vi "Heater_Setpoint_Panel.vi"() -> ()   [LabVIEW 2016]
uses:
  Heater_Setpoint.ctl
  ADAM Controls/Channel_names.ctl
  ADAM Controls/Update_scan_value.ctl
  ADAM Controls/Channel_State.ctl
panel:
  in  "Mode":u16(ring) items=["Only Show Setpoints Above 2 Deg C", "Show all Setpoints"]
  in  "Setpoints Out":T1[](array[typedef])
  out "Messages":string
  in  "OK":bool
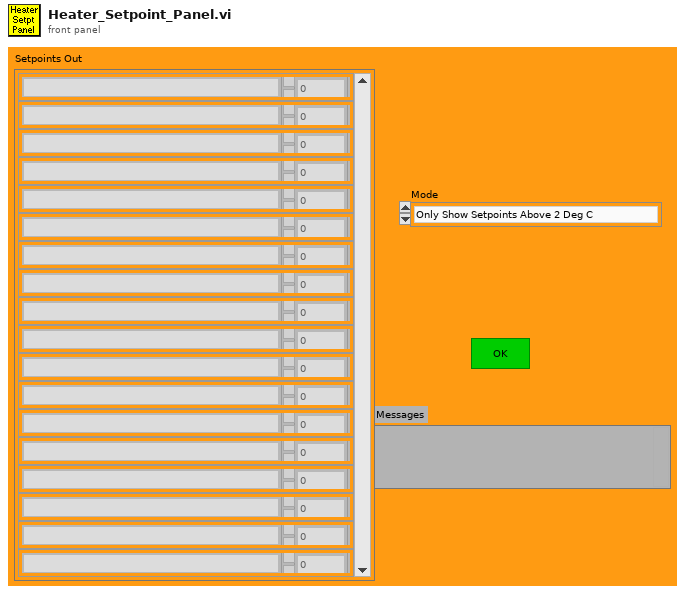
[diagram p1: front panel]
types:
  T1 = typedef "Heater_Setpoint.ctl" = cluster{"Ch Name":string, "Setpoint":dbl}
  T2 = typedef "Channel_names.ctl" = enum16{"Active Only", "Active + Off", "All Channels"}
  T3 = typedef "Update_scan_value.ctl" = cluster{"Channel Name":string, "New Value":dbl}
  T4 = typedef "Channel_State.ctl" = enum16{"On", "Off", "Always On", "Always Off"}
  T5 = typedef "Ch_description_ADAM.ctl" = cluster{"Ch Name":string, "Type":T6, "Function":T7, "Ch State":T4, "Calibration type":T8, "A":dbl, "B":dbl, "C":dbl, "D":dbl, "Comments":string, "Address":T9, "String":string, "Duty":u16}
  T6 = typedef "Module_type_ADAM.ctl" = string
  T7 = typedef "Function_ADAM.ctl" = enum16{"Analogue Input", "Digital Input", "Event counter", "Event rate", "Analogue Output", "Digital Output", "Relay Output"}
  T8 = typedef "Calib_type_ADAM.ctl" = enum16{"Raw", "Bx + A", "Cx^2 + Bx + A", "Dx^3 + Cx^2 + Bx + A", "In Band", "Hi-Tec Q", "Hi-Tec M_dot", "Text"}
  T9 = typedef "Address.ctl" = cluster{"Main":i32, "Ch.":i32, "Sub":i32, "Port Name":string}
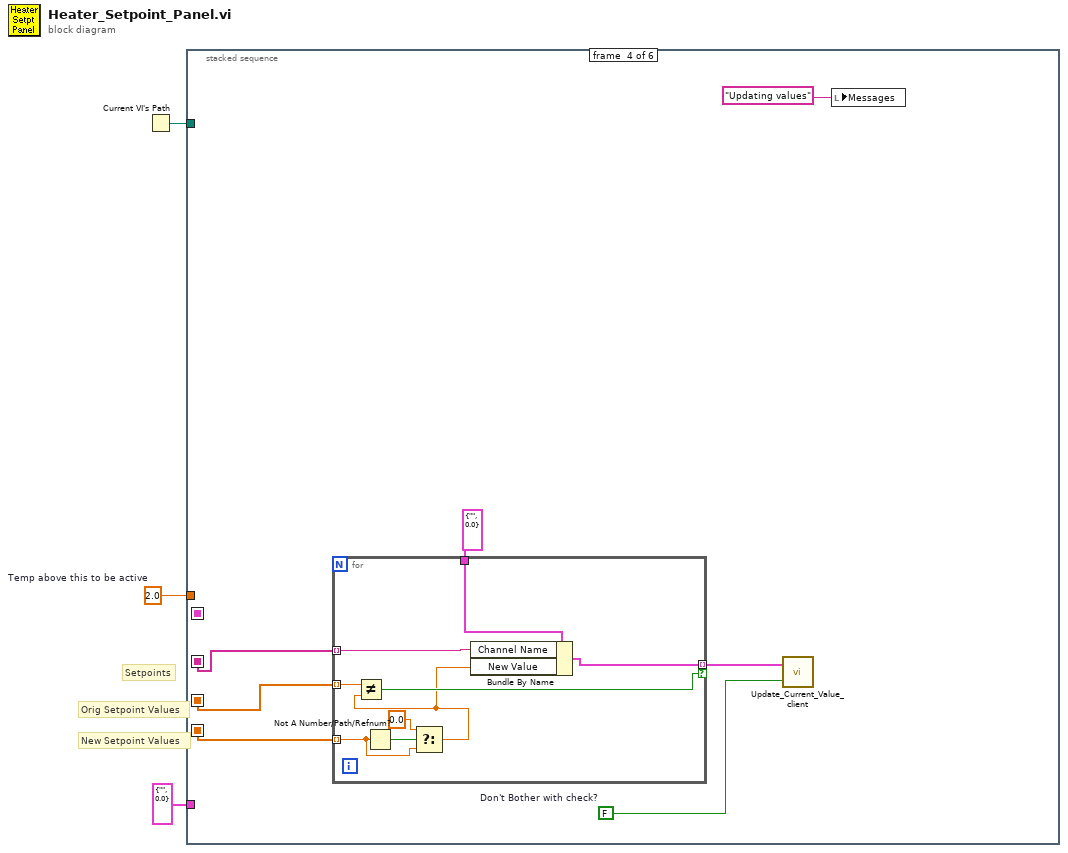
[diagram p0: block diagram]
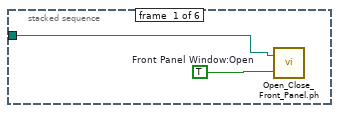
[diagram p2: hidden frame]
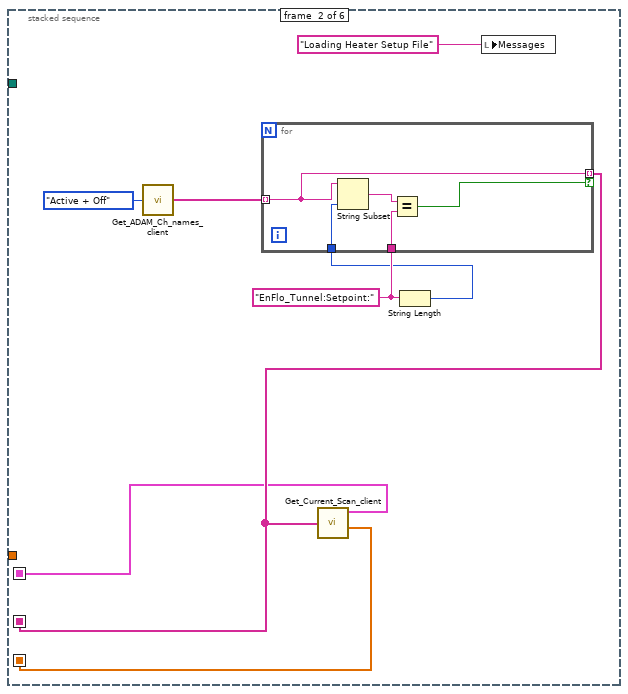
[diagram p3: hidden frame]
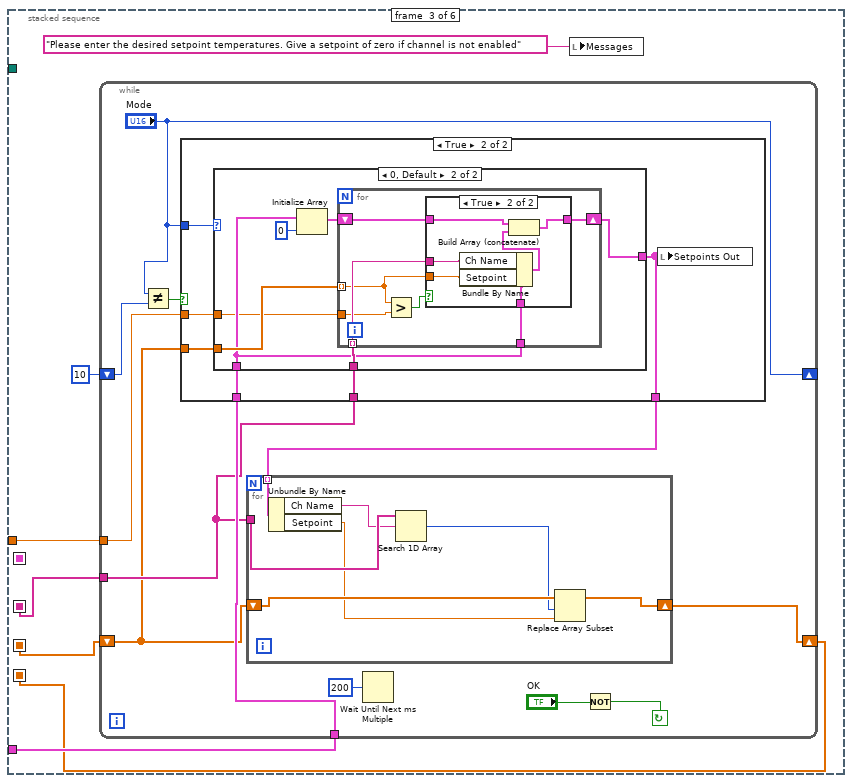
[diagram p4: hidden frame]
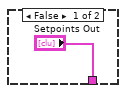
[diagram p5: hidden frame]
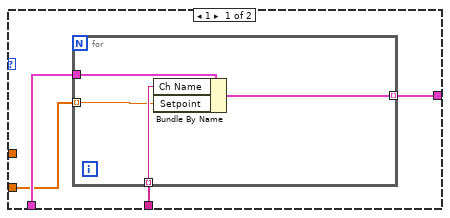
[diagram p6: hidden frame]
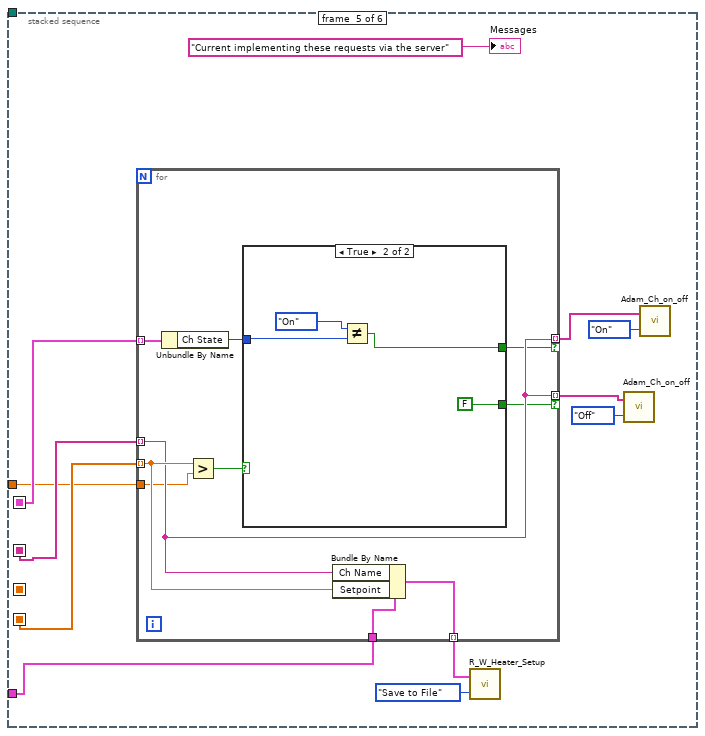
[diagram p8: hidden frame]
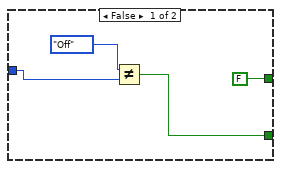
[diagram p9: hidden frame]
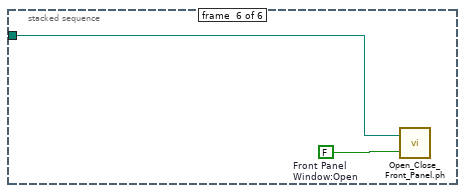
[diagram p10: hidden frame]
diagram:
  w1 = 2.0  # Temp above this to be active
  # "New Setpoint Values"
  # "Orig Setpoint Values"
  # "Setpoints"
  n1 = Current VI's Path() -> (path=w3:path)
  n2 = stacked-sequence {
    seq-local: [_ w8 _ _ _ _] -> [_ _ w22 w82 _ _]
    seq-local: [_ w7 _ _ _ _] -> [_ _ w24 w85 w105 _]
    seq-local: [_ _ w20 _ _ _] -> [_ _ _ w84 w104 _]
    seq-local: [_ w6 _ _ _ _] -> [_ _ _ _ w98 _]
    tunnel: w3 -> [w5 _ _ _ _ w127]
    tunnel: T1 {"Ch Name"="", "Setpoint"=0.0} ("Cluster") -> [_ _ w23 _ w103 _]
    tunnel: w1 -> [_ _ w19 _ w97 _]
    frame #0 {
      w4 = TRUE  # Front Panel Window:Open
      n3 = call "Open_Close_Front_Panel.ph.vi"("Front Panel Window:Open"=w4, "VI path"=w5) -> ()  [unwired: 2 out]
    }
    frame #1 {
      w12 = "EnFlo_Tunnel:Setpoint:"
      n4 = call "Get_ADAM_Ch_names_client.vi"("Channel names set"=Channel_names."Active + Off") -> ("Ch names"=w9:string[])
      n5 = String Length(string=w12) -> (length=w11:i32)
      n6 = for {
        tunnel: w9 -> [w15] mode=indexing
        tunnel: w11 -> [w18]
        tunnel: w12 -> [w17]
        tunnel: [w15] -> w7 mode=indexing if=w14
        n7 = String Subset(string=w15, length (rest)=w18) -> (substring=w16:string)  [unwired: 1 out]
        n8 = Equal?(x=w16, y=w17) -> (x = y?=w14:bool)
      }
      n9 = call "Get_Current_Scan_client.vi"("ADAM Ch Names"=w7) -> ("Ch Description Array"=w6:T5[], "Numerical Values"=w8:dbl[])  [unwired: 2 out]
      n10 = local write "Messages"("Loading Heater Setup File" ("Messages")) -> ()
    }
    frame #2 {
      n11 = while {
        tunnel: w24 -> [w29]
        tunnel: w23 -> [w30]
        shift-right: [w34] -> w20
        shift-left: w22 -> [w28]
        shift-right: ["Mode"] -> _
        shift-left: u16 10 ("Mode") -> [w33]
        tunnel: w19 -> [w26]
        stop <- w36 continue-if-true
        n12 = Not Equal?(x="Mode", y=w33) -> (x != y?=w32:bool)
        n13 = case shown="True" w32 {
          tunnel: "Mode" -> [_ w44]
          tunnel: w30 -> [_ w43]
          tunnel: w29 -> [_ w42]
          tunnel: w28 -> [_ w41]
          tunnel: ["Setpoints Out" w40] -> w27
          tunnel: w26 -> [_ w39]
          frame False {
          }
          frame True {
            n14 = case shown="0, Default" w44 {
              tunnel: w43 -> [w48 w56]
              tunnel: w42 -> [w47 w58]
              tunnel: w41 -> [w46 w59]
              tunnel: [w45 w57] -> w40
              tunnel: w39 -> [_ w53]
              frame 1 {
                n15 = for {
                  tunnel: w48 -> [w52]
                  tunnel: w47 -> [w51] mode=indexing
                  tunnel: w46 -> [w50] mode=indexing
                  tunnel: [w49] -> w45 mode=indexing
                  n16 = Bundle By Name(cluster=w52, "Ch Name"=w51, "Setpoint"=w50) -> (w49:T1)
                }
              }
              frame 0, Default {
                n17 = Initialize Array(w56, 0 ("dimension size")) -> (w54:T1[])
                n18 = for {
                  tunnel: w58 -> [w66] mode=indexing
                  tunnel: w59 -> [w65] mode=indexing
                  tunnel: w56 -> [w63]
                  shift-right: [w62] -> w57
                  shift-left: w54 -> [w61]
                  tunnel: w53 -> [w60]
                  n19 = Greater?(x=w65, y=w60) -> (0:w64:bool)
                  n20 = case shown="True" w64 {
                    tunnel: w66 -> [_ w73]
                    tunnel: w65 -> [_ w72]
                    tunnel: w63 -> [_ w71]
                    tunnel: [w67 w69] -> w62
                    tunnel: w61 -> [w67 w68]
                    frame False {
                    }
                    frame True {
                      n21 = Bundle By Name(cluster=w71, "Ch Name"=w73, "Setpoint"=w72) -> (w70:T1)
                      n22 = Build Array (concatenate)(w68, w70) -> (w69:T1[])
                    }
                  }
                }
              }
            }
            n23 = local write "Setpoints Out"(w40) -> ()
          }
        }
        n24 = for {
          tunnel: w29 -> [w80]
          shift-right: [w77] -> w34
          shift-left: w28 -> [w78]
          tunnel: w27 -> [w74] mode=indexing
          n25 = Unbundle By Name(w74) -> ("Ch Name"=w79:string, "Setpoint"=w75:dbl)
          n26 = Search 1D Array(1D array=w80, element=w79) -> (index of element=w76:i32)  [unwired: 1 out]
          n27 = Replace Array Subset(array=w78, new element=w75, index=w76) -> (w77:dbl[])
        }
        n28 = Wait Until Next ms Multiple(millisecond multiple=u32 200) -> ()  [unwired: 1 out]
        n29 = Not(x="OK") -> (.not. x?=w36:bool)
      }
      n30 = local write "Messages"("Please enter the desired setpoint temperatures. Give a setpoint of zero if channel is not enabled" ("Messages")) -> ()
    }
    frame #3 {
      w83 = FALSE  # Don't Bother with check?
      n31 = for {
        tunnel: T3 {"Channel Name"="", "New Value"=0.0} ("Update Scan Value Cluster") -> [w96]
        tunnel: w85 -> [w95] mode=indexing
        tunnel: w84 -> [w90] mode=indexing
        tunnel: w82 -> [w94] mode=indexing
        tunnel: [w93] -> w81 mode=indexing if=w92
        n32 = Not A Number/Path/Refnum?(number/path/refnum=w90) -> (NaN/Path/Refnum?=w91:bool)
        n33 = Select(t=0.0, s=w91, f=w90) -> (s? t:f=w88:dbl)
        n34 = Not Equal?(x=w94, y=w88) -> (x != y?=w92:bool)
        n35 = Bundle By Name(cluster=w96, "Channel Name"=w95, "New Value"=w88) -> (w93:T3)
      }
      n36 = call "Update_Current_Value_client.vi"("Don't Bother with check?"=w83, "Update array in"=w81) -> ()
      n37 = local write "Messages"("Updating values" ("Messages")) -> ()
    }
    frame #4 {
      n38 = for {
        tunnel: w105 -> [w115] mode=indexing
        tunnel: w104 -> [w116] mode=indexing
        tunnel: w103 -> [w118]
        tunnel: [w117] -> w102 mode=indexing
        tunnel: [w115] -> w100 mode=indexing if=w114
        tunnel: [w115] -> w99 mode=indexing if=w113
        tunnel: w98 -> [w112] mode=indexing
        tunnel: w97 -> [w109]
        n39 = Unbundle By Name(w112) -> ("Ch State"=w110:T4)
        n40 = Greater?(x=w116, y=w109) -> (0:w111:bool)
        n41 = case shown="True" w111 {
          tunnel: [FALSE w124] -> w114
          tunnel: [w119 FALSE] -> w113
          tunnel: w110 -> [w121 w125]
          frame False {
            n42 = Not Equal?(x=Channel_State."Off" ("Ch State"), y=w121) -> (x != y?=w119:bool)
          }
          frame True {
            n43 = Not Equal?(x=Channel_State."On" ("Ch State"), y=w125) -> (x != y?=w124:bool)
          }
        }
        n44 = Bundle By Name(cluster=w118, "Ch Name"=w115, "Setpoint"=w116) -> (w117:T1)
      }
      n45 = call "R_W_Heater_Setup.vi"("Mode"=enum16{"Load from File", "Save to File"}."Save to File", "Setpoints In"=w102) -> ()  [unwired: 2 out]
      n46 = call "Adam_Ch_on_off.vi"("Ch State"=Channel_State."Off", "ADAM Ch Names"=w99) -> ()  [unwired: 1 out]
      n47 = call "Adam_Ch_on_off.vi"("Ch State"=Channel_State."On", "ADAM Ch Names"=w100) -> ()  [unwired: 1 out]
      "Messages" <- "Current implementing these requests via the server" ("Messages")
    }
    frame #5 {
      w128 = FALSE  # Front Panel Window:Open
      n48 = call "Open_Close_Front_Panel.ph.vi"("Front Panel Window:Open"=w128, "VI path"=w127) -> ()  [unwired: 2 out]
    }
  }
